vi "Query Questionable Data Register.vi"(8 "error in (no error)":errorcluster, 11 "VISA resource name":refnum<visa-resource-name>) -> (0 "error out":errorcluster, 1 "Questionable Data Message":string, 3 "VISA resource name out":refnum<visa-resource-name>)   [LabVIEW 2021, in "Agilent 34420.lvlib"]
doc: "Queries the event register for the Questionable Data Register group. Essentially, it is used to observe possible invalid results. For example, if the set sample interval is less than the minimum sample interval, the questionable data register will be set. This VI will then return the corresponding warning(s)."
uses:
  <instrlib>/Agilent 34420/Agilent 34420.lvlib
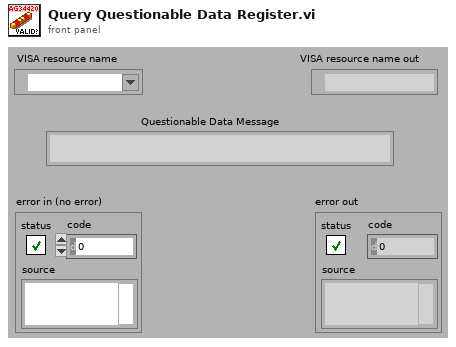
[diagram p1: front panel]
types:
  T1 = cluster{"Boolean array[0]":bool, "Boolean array[1]":bool, "Boolean array[2]":bool, "Boolean array[3]":bool, "Boolean array[4]":bool, "Boolean array[5]":bool, "Boolean array[6]":bool, "Boolean array[7]":bool, "Boolean array[8]":bool, "Boolean array[9]":bool, "Boolean array[10]":bool, "Boolean array[11]":bool, "Boolean array[12]":bool, "Boolean array[13]":bool, "Boolean array[14]":bool, "Boolean array[15]":bool}
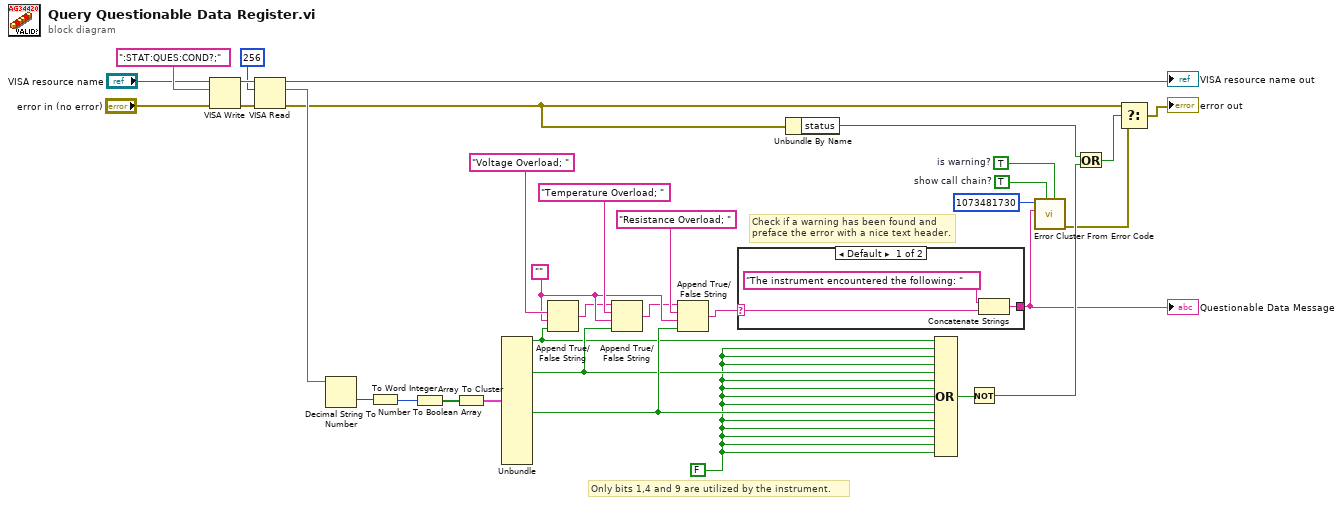
[diagram p0: block diagram]
diagram:
  w7 = TRUE  # is warning?
  w8 = TRUE  # show call chain?
  w1 = FALSE
  w22 = ""
  # "Check if a warning has been found and preface the error with a nice text header."
  # "Only bits 1,4 and 9 are utilized by the instrument."
  n1 = VISA Write(VISA resource name="VISA resource name", write buffer=":STAT:QUES:COND?;", error in (no error)="error in (no error)") -> (VISA resource name out=w32:refnum<visa-resource-name>, error out=w33:errorcluster)  [unwired: 1 out]
  n2 = VISA Read(VISA resource name=w32, byte count=u32 256, error in (no error)=w33) -> (VISA resource name out=→"VISA resource name out":refnum<visa-resource-name>, read buffer=w30:string, error out=w11:errorcluster)  [unwired: 1 out]
  n3 = Decimal String To Number(string=w30) -> (number=w27:i32)  [unwired: 2 in, 1 out]
  n4 = To Word Integer(number=w27) -> (16bit integer=w28:i16)
  n5 = Number To Boolean Array(number=w28) -> (Boolean array=w29:bool[])
  n6 = Array To Cluster(array=w29) -> (cluster=w26:T1)
  n7 = Unbundle(w26) -> ("Boolean array[0]"=w17:bool, "Boolean array[4]"=w18:bool, "Boolean array[9]"=w19:bool)  [unwired: 13 out]
  n8 = Append True/False String(1:w17, 2:w22, 3:"Voltage Overload; " ("true string")) -> (0:w3:string)  [unwired: 1 in]
  n9 = Append True/False String(1:w18, 2:w22, 3:"Temperature Overload; " ("true string"), 4:w3) -> (0:w2:string)
  n10 = Append True/False String(1:w19, 2:w22, 3:"Resistance Overload; " ("true string"), 4:w2) -> (0:w4:string)
  n11 = case shown="Default" w4 {
    selector: w4 -> [w36 w38]
    tunnel: [w35 w38] -> w5
    frame Default {
      n12 = Concatenate Strings("The instrument encountered the following: " ("true string"), w36) -> (w35:string)
    }
    frame "" {
    }
  }
  "Questionable Data Message" <- w5
  n13 = Unbundle By Name(w11) -> ("status"=w14:bool)
  n14 = Compound Arithmetic op=OR(w17, w1, w1, w1, w18, w1, w1, w1, w1, w19, w1, w1, w1, w1, w1) -> (w16:bool)
  n15 = Not(x=w16) -> (.not. x?=w15:bool)
  n16 = call <vilib>:"Error Cluster From Error Code.vi"("is warning? (False)"=w7, "show call chain? (False)"=w8, "error message (\"\")"=w5, "error code (0)"=1073481730 ("t")) -> ("error out"=w10:errorcluster)  [unwired: 5 in]
  n17 = Or(x=w14, y=w15) -> (x .or. y?=w13:bool)
  n18 = Select(t=w11, s=w13, f=w10) -> (s? t:f=→"error out":errorcluster)
